vi "ConfigFileBackup.vi"(9 "CurrentVIPath":path, 11 "ConfigFilePath":path) -> (1 "Success?":bool)   [LabVIEW 2017]
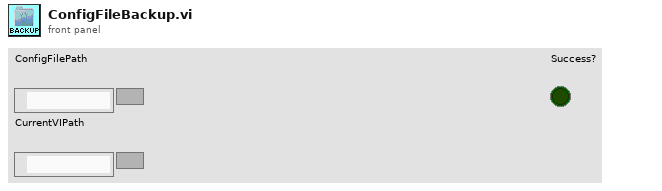
[diagram p1: front panel]
types:
  T1 = enum16{"open", "replace", "create", "open or create", "replace or create", "replace or create with confirmation"}
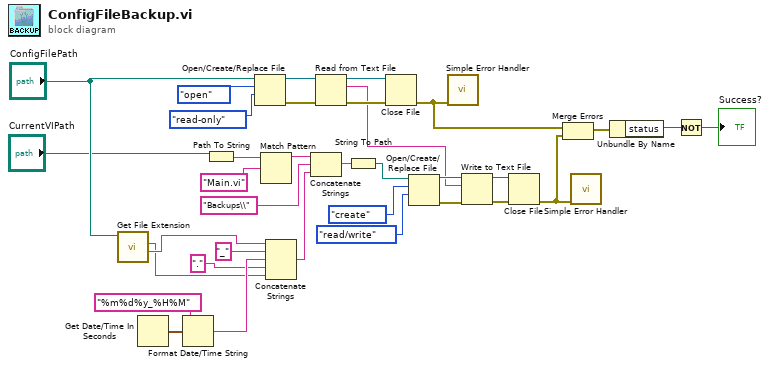
[diagram p0: block diagram]
diagram:
  n1 = call <vilib>:"Get File Extension.vi"("file"="ConfigFilePath") -> ("filename without extension"=w10:string, "lowercase file extension"=w9:string)  [unwired: 6 in, 3 out]
  n2 = Get Date/Time In Seconds() -> (seconds since 1Jan1904=w29:timestamp)
  n3 = Format Date/Time String(time format string (%c)="%m%d%y_%H%M", seconds (now)=w29) -> (date/time string=w27:string)  [unwired: 1 in]
  n4 = Path To String(path="CurrentVIPath") -> (string=w34:string)
  n5 = Open/Create/Replace File(file path (use dialog)="ConfigFilePath", operation (0:open)=T1."open", access (0:read/write)=enum16{"read/write", "read-only", "write-only"}."read-only") -> (refnum out=w23:refnum<file>, error out=w24:errorcluster)  [unwired: 3 in, 1 out]
  n6 = Match Pattern(string=w34, regular expression="Main.vi") -> (before substring=w32:string)  [unwired: 1 in, 3 out]
  n7 = Concatenate Strings(w10, "_", w27, ".", w9) -> (w15:string)
  n8 = Concatenate Strings(w32, "Backups\\", w15) -> (w14:string)
  n9 = Read from Text File(file (use dialog)=w23, error in=w24) -> (refnum out=w21:refnum<file>, text=w16:string, error out=w22:errorcluster)  [unwired: 2 in, 1 out]
  n10 = String To Path(string=w14) -> (path=w13:path)
  n11 = Close File(refnum=w21, error in=w22) -> (error out=w4:errorcluster)  [unwired: 1 out]
  n12 = Open/Create/Replace File(file path (use dialog)=w13, operation (0:open)=T1."create", access (0:read/write)=enum16{"read/write", "read-only", "write-only"}."read/write") -> (refnum out=w17:refnum<file>, error out=w18:errorcluster)  [unwired: 3 in, 1 out]
  n13 = call <vilib>:"Simple Error Handler.vi"("error in (no error)"=w4) -> ()  [unwired: 4 in, 5 out]
  n14 = Write to Text File(file (use dialog)=w17, text=w16, error in=w18) -> (refnum out=w11:refnum<file>, error out=w12:errorcluster)  [unwired: 1 in, 1 out]
  n15 = Close File(refnum=w11, error in=w12) -> (error out=w5:errorcluster)  [unwired: 1 out]
  n16 = Merge Errors(w4, w5) -> (w3:errorcluster)
  n17 = call <vilib>:"Simple Error Handler.vi"("error in (no error)"=w5) -> ()  [unwired: 4 in, 5 out]
  n18 = Unbundle By Name(w3) -> ("status"=w2:bool)
  n19 = Not(x=w2) -> (.not. x?=→"Success?":bool)
